vi "poops.vi"(1 "enabled?":bool) -> ()   [LabVIEW 2012]
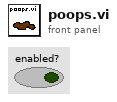
[diagram p1: front panel]
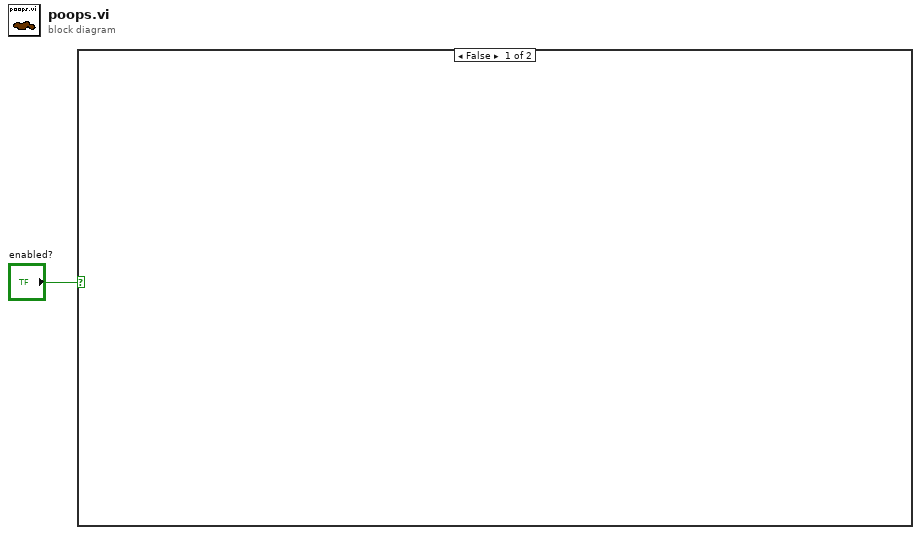
[diagram p0: block diagram]
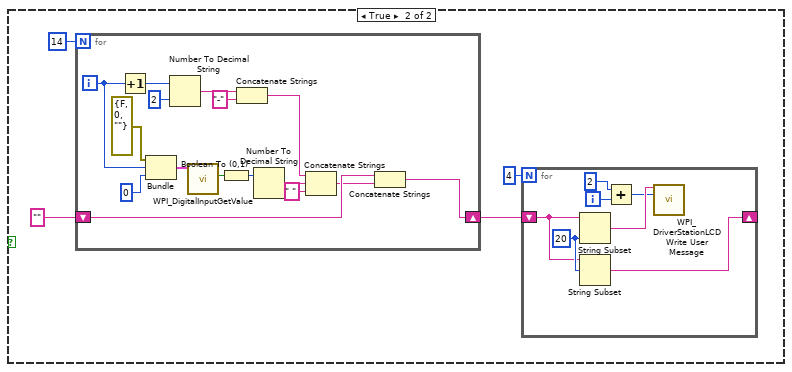
[diagram p2: hidden frame]
diagram:
  n1 = case shown="False" "enabled?" {
    frame False {
    }
    frame True {
      n2 = for {
        N: 14 -> [_]
        shift-right: [w18] -> w3
        shift-left: "" ("string") -> [w20]
        i -> [w17]
        n3 = Increment(x=w17) -> (x+1=w16:i32)
        n4 = Bundle("DevStatus"=errorcluster {"status"=FALSE, "code"=0, "source"=""}, w17, 0) -> (w13:cluster{"DevStatus":errorcluster, i32, i32})  [unwired: 1 in]
        n5 = Number To Decimal String(number=w16, width (-)=i16 2) -> (decimal integer string=w24:string)
        n6 = call <vilib>:"WPI_DigitalInputGetValue.vi"("DigitalInputDevRef"=w13) -> ("Value"=w14:bool)  [unwired: 8 in, 2 out]
        n7 = Boolean To (0,1)(Boolean=w14) -> (0, 1=w26:i16)
        n8 = Concatenate Strings(w24, "-" ("string")) -> (w22:string)
        n9 = Number To Decimal String(number=w26) -> (decimal integer string=w25:string)  [unwired: 1 in]
        n10 = Concatenate Strings(w22, w25, " " ("string")) -> (w19:string)
        n11 = Concatenate Strings(w20, w19) -> (w18:string)
      }
      n12 = for {
        N: 4 -> [_]
        shift-right: [w10] -> _
        shift-left: w3 -> [w11]
        i -> [w8]
        w12 = 20 ("length (rest)")
        n13 = String Subset(string=w11, length (rest)=w12) -> (substring=w9:string)  [unwired: 1 in]
        n14 = String Subset(string=w11, offset (0)=w12) -> (substring=w10:string)  [unwired: 1 in]
        n15 = Add(x=2, y=w8) -> (x+y=w6:i32)
        n16 = call <vilib>:"WPI_DriverStationLCDWrite User Message.vi"("line text"=w9, "line"=w6) -> ()  [unwired: 13 in, 1 out]
      }
    }
  }
